vi "sv_Convert Time Segment to Index.vi"(0 "sampling frequency [Hz]":dbl=10000.0 format="%.2f", 1 "array size":i32, 2 "FFT block size":i32=1024 min=1, 3 "time segment":T1={"from [s]"=-1.0, "to [s]"=-1.0, "time increment"=100.0, "time increment units (%)"=enum."%"} {"time increment" format="%.2f"; "to [s]" format="%.2f"; "from [s]" format="%.2f"}) -> (5 "FFT info":T2={"FFT block size"=1024, "number of FFT"=0, "start index"=0, "increment"=0.0} {"increment" format="%.2f"}, 6 "to and delta t [s]":cluster{"to":dbl, "delta t":dbl} {"delta t" format="%.2f"; "to" format="%.2f"})   [LabVIEW 2017, in "SoundVib_Transient.lvlib"]
uses:
  <vilib>/addons/Sound and Vibration/svt_Transients/SoundVib_Transient.lvlib
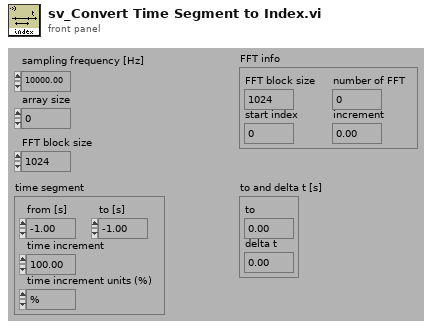
[diagram p1: front panel]
types:
  T1 = cluster{"from [s]":dbl, "to [s]":dbl, "time increment":dbl, "time increment units (%)":enum16{"%", "s", "ms"}}
  T2 = cluster{"FFT block size":i32, "number of FFT":i32, "start index":i32, "increment":dbl}
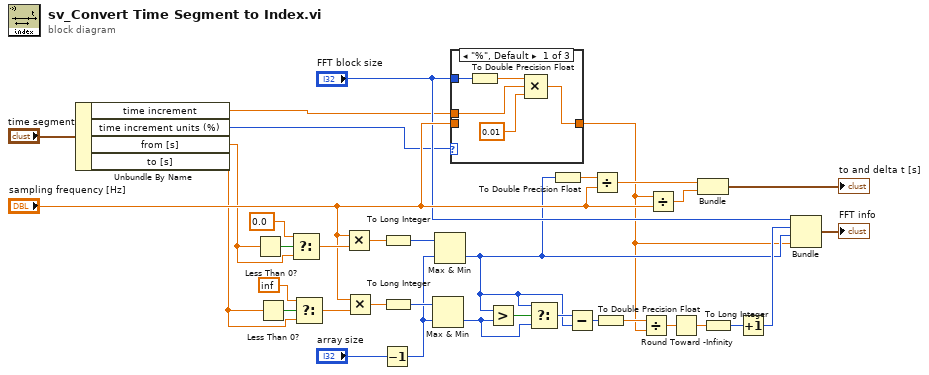
[diagram p0: block diagram]
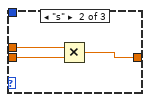
[diagram p2: hidden frame]
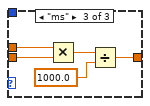
[diagram p3: hidden frame]
diagram:
  n1 = Unbundle By Name("time segment") -> ("time increment"=w4:dbl, "time increment units (%)"=w3:enum16{"%", "s", "ms"}, "from [s]"=w2:dbl, "to [s]"=w1:dbl)
  n2 = Less Than 0?(x=w2) -> (x < 0?=w34:bool)
  n3 = Less Than 0?(x=w1) -> (x < 0?=w32:bool)
  n4 = Select(t=0.0, s=w34, f=w2) -> (s? t:f=w29:dbl)
  n5 = Select(t=inf, s=w32, f=w1) -> (s? t:f=w30:dbl)
  n6 = Multiply(x="sampling frequency [Hz]", y=w29) -> (x*y=w33:dbl)
  n7 = Multiply(x="sampling frequency [Hz]", y=w30) -> (x*y=w28:dbl)
  n8 = Decrement(x="array size") -> (x-1=w25:i32)
  n9 = To Long Integer(number=w33) -> (32bit integer=w26:i32)
  n10 = To Long Integer(number=w28) -> (32bit integer=w27:i32)
  n11 = Max & Min(x=w27, y=w25) -> (min(x,y)=w23:i32)  [unwired: 1 out]
  n12 = Max & Min(x=w26, y=w25) -> (min(x,y)=w8:i32)  [unwired: 1 out]
  n13 = case shown="\"%\", Default" w3 {
    tunnel: w4 -> [w40 w43 w48]
    tunnel: "FFT block size" -> [w37 _ _]
    tunnel: [w36 w41 w44] -> w7
    tunnel: "sampling frequency [Hz]" -> [_ w42 w47]
    frame "%", Default {
      n14 = To Double Precision Float(number=w37) -> (double precision float=w38:dbl)
      n15 = Compound Arithmetic op=MULTIPLY(w38, w40, 0.01 ("y")) -> (w36:dbl)
    }
    frame "s" {
      n16 = Multiply(x=w43, y=w42) -> (x*y=w41:dbl)
    }
    frame "ms" {
      n17 = Multiply(x=w48, y=w47) -> (x*y=w46:dbl)
      n18 = Divide(x=w46, y=1000.0) -> (x/y=w44:dbl)
    }
  }
  n19 = Greater?(x=w8, y=w23) -> (0:w24:bool)
  n20 = Select(t=w8, s=w24, f=w23) -> (s? t:f=w22:i32)
  n21 = To Double Precision Float(number=w8) -> (double precision float=w16:dbl)
  n22 = Subtract(x=w22, y=w8) -> (x-y=w21:i32)
  n23 = Divide(x=w16, y="sampling frequency [Hz]") -> (x/y=w15:dbl)
  n24 = To Double Precision Float(number=w21) -> (double precision float=w20:dbl)
  n25 = Divide(x=w20, y=w7) -> (x/y=w19:dbl)
  n26 = Divide(x=w7, y="sampling frequency [Hz]") -> (x/y=w14:dbl)
  n27 = Round Toward -Infinity(1:w19) -> (0:w18:dbl)
  n28 = Bundle(w15, w14) -> (→"to and delta t [s]":cluster{dbl, dbl})  [unwired: 1 in]
  n29 = To Long Integer(number=w18) -> (32bit integer=w17:i32)
  n30 = Increment(x=w17) -> (x+1=w9:i32)
  n31 = Bundle("FFT block size"="FFT block size", w9, w8, w7) -> (→"FFT info":cluster{"FFT block size":i32, i32, i32, dbl})  [unwired: 1 in]
